vi "motor (SubVI).vi"(0 "VISA Refnum in":refnum<visa-resource-name>, 1 "step":dbl, 3 "error in (no error)":errorcluster) -> (14 "VISA resource name out":refnum<visa-resource-name>, 15 "Angle":dbl, 17 "error out":errorcluster)   [LabVIEW 2014]
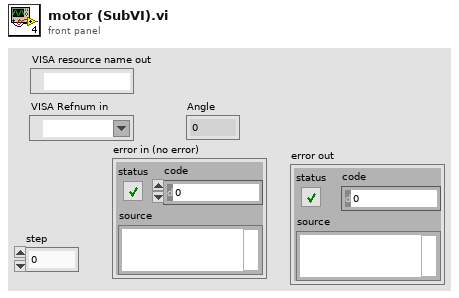
[diagram p1: front panel]
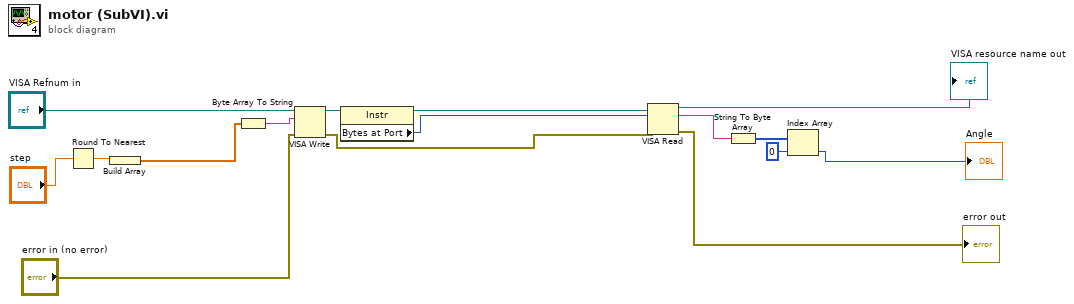
[diagram p0: block diagram]
diagram:
  n1 = Round To Nearest(number="step") -> (nearest integer value=w5:dbl)
  n2 = Build Array(w5) -> (w3:dbl[])
  n3 = Byte Array To String(unsigned byte array=w3) -> (string=w4:string)
  n4 = VISA Write(VISA resource name="VISA Refnum in", write buffer=w4, error in (no error)="error in (no error)") -> (VISA resource name out=w13:refnum<visa-resource-name>, error out=w10:errorcluster)  [unwired: 1 out]
  n5 = property class="Instr"(reference=w13) -> (reference out=w14:refnum<visa-resource-name>, "Bytes at Port"=w15:u32)  [unwired: 1 in, 1 out]
  n6 = VISA Read(VISA resource name=w14, byte count=w15, error in (no error)=w10) -> (VISA resource name out=→"VISA resource name out":refnum<visa-resource-name>, read buffer=w8:string, error out=→"error out":errorcluster)  [unwired: 1 out]
  n7 = String To Byte Array(string=w8) -> (unsigned byte array=w7:u8[])
  n8 = Index Array(array=w7, index=0) -> (element=→"Angle":u8)
